vi "Update Site Lists From BIMS Server.vi"(4 "error IN":errorcluster, 6 "Site":string, 7 "Lookup Table Name":string) -> (0 "error OUT":errorcluster, 3 "recordset data":string[][](array[string]))   [LabVIEW 2015]
uses:
  <vilib>/addons/database/Connection.llb/DB Tools Open Connec (Path).vi
  <vilib>/addons/database/Connection.llb/Conn Execute.vi
  <vilib>/addons/database/Recordset.llb/Rec Destroy - Connection.vi
  <vilib>/addons/database/NI_Database_API.lvlib
panel:
  out "App.Dir":path
  out "SP Call":string
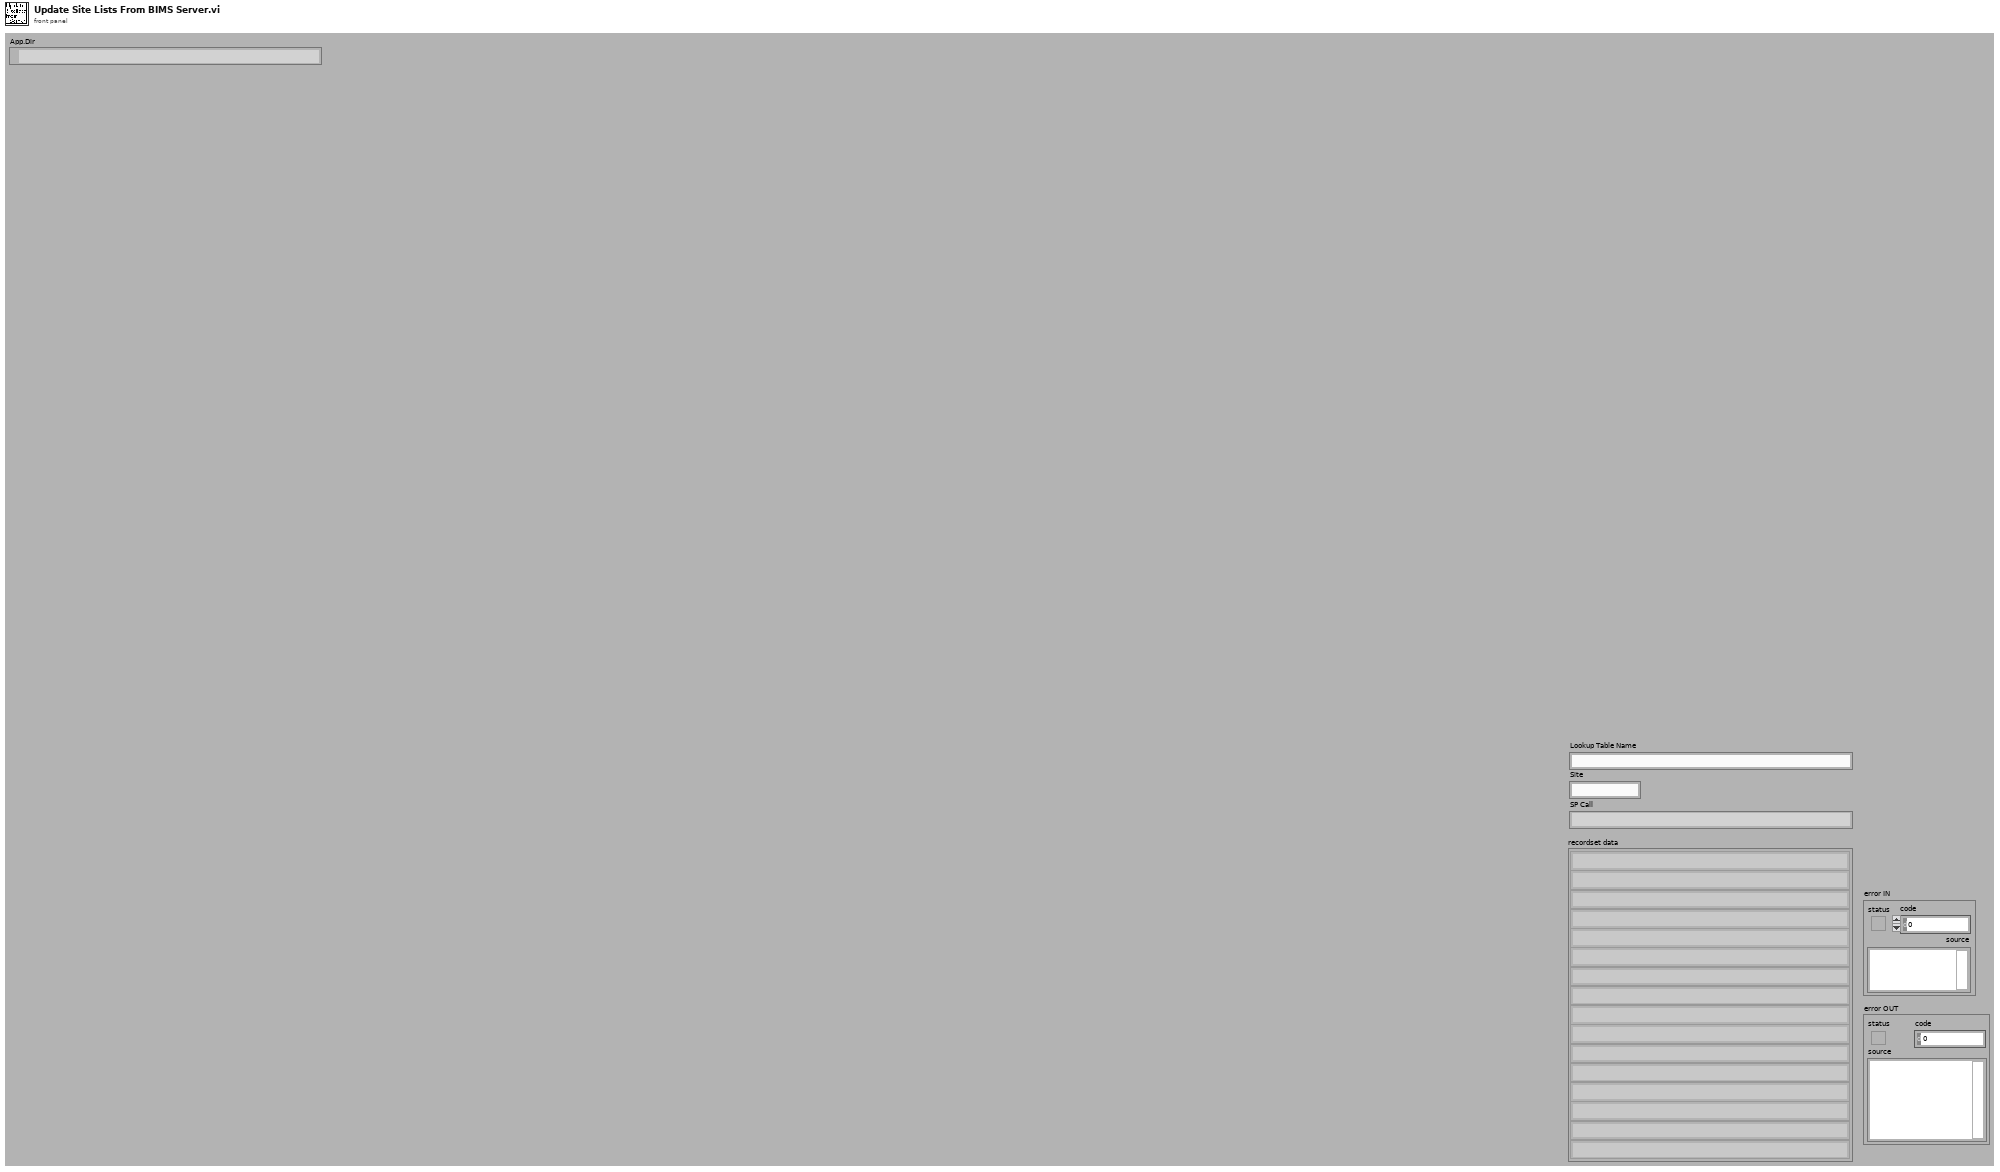
[diagram p1: front panel]
types:
  T1 = enum32{"invalid app kind", "Development System", "Run Time System", "Student Edition", "Embedded LabVIEW", "Evaluation", "Custom"}
  T2 = typedef "NI_Database_API.lvlib/Conn ObjectReference.ctl" = refnum<k1>
  T3 = typedef "NI_Database_API.lvlib/Rec ObjectReference.ctl" = refnum<k1>
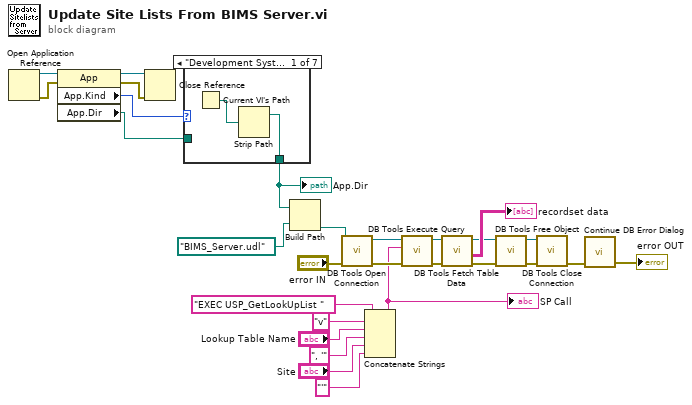
[diagram p0: block diagram]
diagram:
  n1 = Open Application Reference() -> (0:w6:errorcluster, 3:w7:refnum<vi>)  [unwired: 1 in, 3 out]
  n2 = property class="App"(reference=w7, error in=w6) -> (reference out=w5:refnum<vi>, error out=w4:errorcluster, "App.Kind"=w3:T1, "App.Dir"=w2:path)
  n3 = Close Reference(reference=w5, error in (no error)=w4) -> ()  [unwired: 1 out]
  n4 = case shown="\"Development System\"" w3 {
    tunnel: [w29 w31 w32 w33 w34 w35 w36] -> w1
    tunnel: w2 -> [_ w31 w32 w33 w34 w35 w36]
    frame "Development System" {
      n5 = Current VI's Path() -> (path=w30:path)
      n6 = Strip Path(path=w30) -> (stripped path=w29:path)  [unwired: 1 out]
    }
    frame "Run Time System" {
    }
    frame "Student Edition" {
    }
    frame "Embedded LabVIEW" {
    }
    frame "Evaluation" {
    }
    frame "Custom" {
    }
    frame "invalid app kind" {
    }
  }
  "App.Dir" <- w1
  n7 = Build Path(base path=w1, name or relative path=path "BIMS_Server.udl" ("connectString")) -> (appended path=w15:path)
  n8 = call-poly <vilib>:"DB Tools Open Connection.vi"("error in (no error)"="error IN", "connection information"=w15) -> ("error out"=w21:errorcluster, "connection reference"=w19:T2)  [unwired: 3 in, 3 out]
  n9 = Concatenate Strings("EXEC USP_GetLookUpList " ("string"), "v" ("string"), "Lookup Table Name", ", '", "Site", "'") -> (w14:string)
  "SP Call" <- w14
  n10 = call-poly <vilib>:"DB Tools Execute Query.vi"("error in (no error)"=w21, "SQL query"=w14, "connection reference"=w19) -> ("error out"=w22:errorcluster, "recordset reference"=w18:T3)  [unwired: 1 in, 4 out]
  n11 = call <vilib>:"DB Tools Fetch Table Data.vi"("error in (no error)"=w22, "recordset reference"=w18) -> ("error out"=w23:errorcluster, "recordset data"=→"recordset data":string[][], "recordset reference out"=w17:T3)  [unwired: 3 out]
  n12 = call-poly <vilib>:"DB Tools Free Object.vi"("error in (no error)"=w23, "recordset reference"=w17) -> ("error out"=w24:errorcluster, "connection reference"=w20:T2)  [unwired: 8 out]
  n13 = call <vilib>:"DB Tools Close Connection.vi"("error in (no error)"=w24, "connection reference"=w20) -> ("error out"=w26:errorcluster)  [unwired: 5 out]
  n14 = call "Continue DB Error Dialog.vi"("error in (no error)"=w26) -> ("error out"=→"error OUT":errorcluster)  [unwired: 3 in, 2 out]
